vi "Write HttpContent.vi"(8 "error in (no error)":errorcluster, 10 "HttpContent":refnum<class "HttpContent.lvclass">, 11 "HttpRequestMessage in":refnum<class "HttpRequestMessage.lvclass">) -> (0 "error out":errorcluster, 3 "HttpRequestMessage out":refnum<class "HttpRequestMessage.lvclass">)   [LabVIEW 2018, in "HttpClient_NET.lvlib" / "HttpRequestMessage.lvclass"]
doc: "<b> </b> <b> </b>\nHttpClient_NET\nJustin Young - Viviota\nCopyright (c) 2021\nLicense: BSD"
uses:
  HttpRequestMessage.lvclass
  HttpContent/HttpContent.lvclass
  HttpContent/HttpContent.lvclass/HttpContent.ctl
  HttpRequestMessage.lvclass/HttpRequestMessage.ctl
  HttpContent/Accessors/Read NET_HttpContent.vi
  Accessors/Read NET_HttpRequestMessage.vi
  System.Net.Http
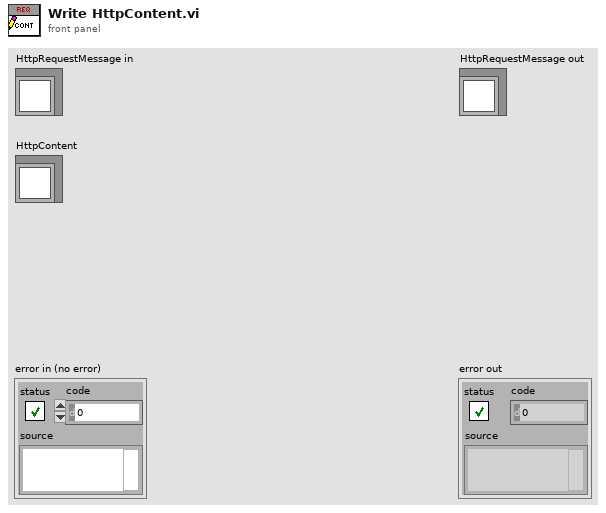
[diagram p1: front panel]
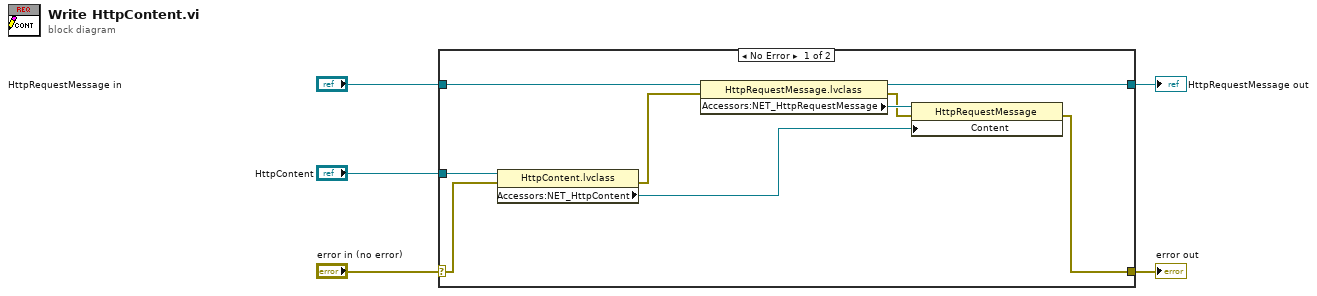
[diagram p0: block diagram]
diagram:
  n1 = case shown="No Error" "error in (no error)" {
    selector: "error in (no error)" -> [w9 w15]
    tunnel: [w6 w15] -> w4
    tunnel: [w10 w16] -> w2
    tunnel: "HttpRequestMessage in" -> [w13 w16]
    tunnel: "HttpContent" -> [w14 _]
    frame No Error {
      n2 = property class="HttpContent.lvclass"(reference=w14, error in=w9) -> (error out=w8:errorcluster, "Accessors:NET_HttpContent"=w11:refnum<k24>)  [unwired: 1 out]
      n3 = property class="HttpRequestMessage.lvclass"(reference=w13, error in=w8) -> (reference out=w10:refnum<class "HttpRequestMessage.lvclass">, error out=w7:errorcluster, "Accessors:NET_HttpRequestMessage"=w12:refnum<k24>)
      n4 = property class="HttpRequestMessage"(reference=w12, error in=w7, "Content"=w11) -> (error out=w6:errorcluster)  [unwired: 1 out]
    }
    frame Error {
    }
  }
  "error out" <- w4
  "HttpRequestMessage out" <- w2
